vi "NML GPIB Data Log V1.00.vi"(0 "Point #":i32) -> (1 "GPIB Data":dbl[](array[numeric]) format="%.2e", 2 "Stop":bool)   [LabVIEW 2021]
doc: "VI which calls the appropriate GPIB routines for a variety of instruments.\nScott Hannahs, NHMFL-FSU, Nov. 1993"
uses:
  GPIB List.ctl
  Sub Controls/Instrument.ctl
  Sub Controls/NML GPIB List.ctl
panel:
  in  "Instrument":T1
  in  "Logcluster":T2 {"#1"."Parameters" format="%.3e"; "#5"."Parameters" format="%.3e"; "#3"."Parameters" format="%.3e"; "#2"."Parameters" format="%.3e"; "#4"."Parameters" format="%.3e"}
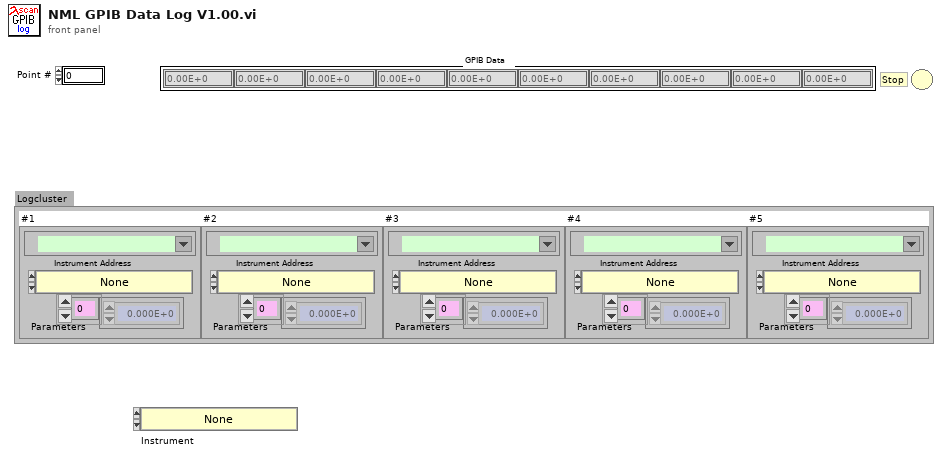
[diagram p1: front panel]
types:
  T1 = typedef "NML GPIB List.ctl" = enum16{"None", "Field", "Field - SCM1", "DMM", "DMM - HP 34401", "Keithley 2XXX", "Running DMM Ave", "Running HP34401", "Running K2XXX Ave", "SRS 830 - CH 1", "SRS 830 - CH1 & 2", "SRS PTC10", "Signal Rec 7265 - X", "Signal Rec 7265 - X&Y", "DRC 93C - Sample", "DRC 93C - Control", "DRC 93C - Sam&Con", "CryoCon Sensor A", "CryoCon Sensor B", "Cond 20C Sensor 1", "Cond 20C Sensor 2", "LS 336 Read", "LS 340 Read", "LS 370 Read", "LS 370 Select", "AVS 46 Bridge", "BLM Rotator Read Position", "Linear Research 700", "LR 700 Select", "Keithley 3330 - LCZ", "A-H Capacitance", "Digital Integrator", "SRS 400 Phot Ctr", "LakeShore VSM", "AMI He Level Meter", "Time Stamp", "Wait", "Invert Current", "K230 Linear V", "K230 VÅB^2", "Temp Ramp", "Power Ramp", "Freq Sweep", "LTC Stable T", "Scanner Step", "IMS Stepper Increment", "BLM Stepper Increment", "Omega CNi32"}
  T2 = typedef "GPIB List.ctl" = cluster{"#4":T3, "#2":T3, "#3":T3, "#5":T3, "#1":T3}
  T3 = typedef "Instrument.ctl" = cluster{"Instrument":T1, "Instrument Address":refnum<visa-resource-name>, "Parameters":dbl[]}
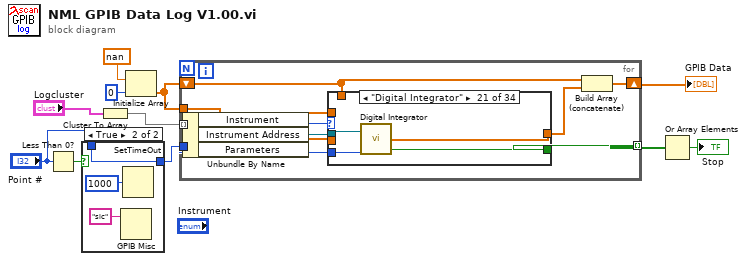
[diagram p0: block diagram]
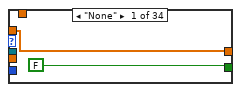
[diagram p3: hidden frame]
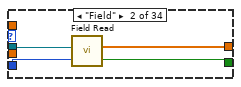
[diagram p4: hidden frame]
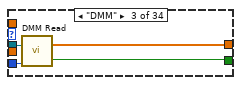
[diagram p5: hidden frame]
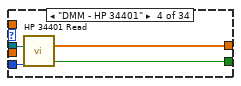
[diagram p6: hidden frame]
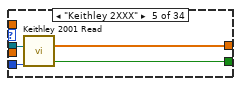
[diagram p7: hidden frame]
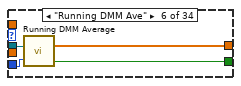
[diagram p8: hidden frame]
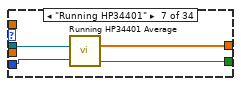
[diagram p9: hidden frame]
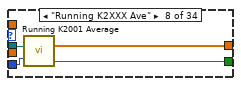
[diagram p10: hidden frame]
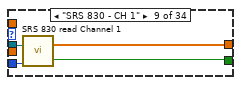
[diagram p11: hidden frame]
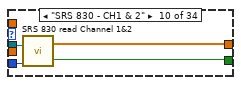
[diagram p12: hidden frame]
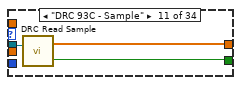
[diagram p13: hidden frame]
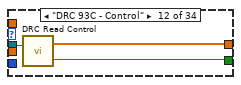
[diagram p14: hidden frame]
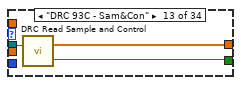
[diagram p15: hidden frame]
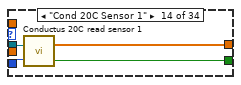
[diagram p16: hidden frame]
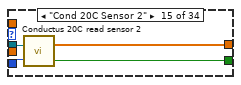
[diagram p17: hidden frame]
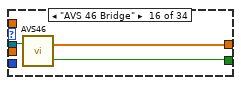
[diagram p18: hidden frame]
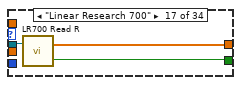
[diagram p19: hidden frame]
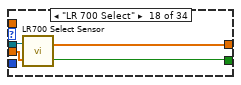
[diagram p20: hidden frame]
diagram:
  n1 = Less Than 0?(x="Point #") -> (x < 0?=w5:bool)
  n2 = case shown="True" w5 {
    tunnel: [w12 w14] -> w3
    tunnel: "Point #" -> [w12 w14]
    frame False {
    }
    frame True {
      n3 = GPIB Misc(0:"sic" ("command string")) -> ()  [unwired: 1 in, 3 out]
      n4 = SetTimeOut(1:1000 ("new timeout (10000)")) -> ()  [unwired: 1 out]
    }
  }
  n5 = Cluster To Array(cluster="Logcluster") -> (array=w1:T3[])
  n6 = Initialize Array(nan, 0) -> (w7:dbl[])
  n7 = for {
    shift-right: [w25] -> w11
    shift-left: w7 -> [w20]
    tunnel: w3 -> [w23]
    tunnel: [w22] -> w6 mode=indexing
    tunnel: w7 -> [w21]
    tunnel: w1 -> [w19] mode=indexing
    n8 = Unbundle By Name(w19) -> ("Instrument"=w16:T1, "Instrument Address"=w18:refnum<visa-resource-name>, "Parameters"=w17:dbl[])
    n9 = case shown="\"Digital Integrator\"" w16 {
      tunnel: [FALSE w30 w34 w38 w42 w46 w50 w54 w59 w63 w66 w69 w72 w75 w79 w82 w85 w89 w92 w96 w98 w104 w107 w109 w113 w118 w123 w128 w133 w138 w140 w146 w152 w154] -> w22
      tunnel: w23 -> [_ w28 w32 w36 w40 w44 w48 w52 w56 w60 _ _ _ w73 w77 _ _ _ _ w94 w101 _ _ w111 w115 w116 w120 w126 w131 w136 w142 w147 w151 w158]
      tunnel: [w26 w31 w35 w39 w43 w47 w51 w55 w58 w62 w65 w68 w71 w76 w80 w81 w84 w88 w91 w95 w99 w105 w108 w110 w114 w119 w124 w129 w134 w139 w141 w145 w153 w155] -> w24
      tunnel: w18 -> [_ w29 w33 w37 w41 w45 w49 w53 w57 w61 w64 w67 w70 w74 w78 w83 w86 w90 w93 w97 w100 w103 w106 _ _ w117 w122 w127 w132 w137 w143 w148 w150 w156]
      tunnel: w21 -> [w26 _ _ _ _ _ _ _ _ _ _ _ _ _ _ _ _ _ _ _ _ _ _ _ _ _ _ _ _ _ _ _ _ _]
      tunnel: w17 -> [_ _ _ _ _ _ _ _ _ _ _ _ _ _ _ _ _ w87 _ _ _ w102 _ _ w112 _ w121 _ w130 w135 _ w144 w149 w157]
      tunnel: w20 -> [_ _ _ _ _ _ _ _ _ _ _ _ _ _ _ _ _ _ _ _ _ _ _ _ _ _ _ w125 _ _ _ _ _ _]
      frame "None" {
      }
      frame "Field" {
        n10 = call "Field Read.vi"("Point #"=w28, "Instrument Address"=w29) -> ("Stop"=w30:bool, "Field"=w31:dbl[])
      }
      frame "DMM" {
        n11 = call "DMM Read.vi"("Point #"=w32, "Instrument Address"=w33) -> ("Stop"=w34:bool, "Measurement"=w35:dbl[])
      }
      frame "DMM - HP 34401" {
        n12 = call "HP 34401 Read.vi"("Point #"=w36, "Instrument Address"=w37) -> ("Stop"=w38:bool, "Measurement"=w39:dbl[])
      }
      frame "Keithley 2XXX" {
        n13 = call "Keithley 2001 Read.vi"("Point #"=w40, "Instrument Address"=w41) -> ("Stop"=w42:bool, "Measurement"=w43:dbl[])
      }
      frame "Running DMM Ave" {
        n14 = call "Running DMM Average.vi"("Point #"=w44, "Instrument Address"=w45) -> ("Stop"=w46:bool, 1:w47:dbl[])
      }
      frame "Running HP34401" {
        n15 = call "Running HP34401 Average.vi"("Point #"=w48, "Instrument Address"=w49) -> ("Stop"=w50:bool, 1:w51:dbl[])
      }
      frame "Running K2XXX Ave" {
        n16 = call "Running K2001 Average.vi"("Point #"=w52, "Instrument Address"=w53) -> ("Stop"=w54:bool, 1:w55:dbl[])
      }
      frame "SRS 830 - CH 1" {
        n17 = call "SRS 830 read Channel 1.vi"("Point #"=w56, "Instrument Address"=w57) -> ("Stop"=w59:bool, "SRS 830 Output"=w58:dbl[])
      }
      frame "SRS 830 - CH1 & 2" {
        n18 = call "SRS 830 read Channel 1&2.vi"("Point #"=w60, "Instrument Address"=w61) -> ("Stop"=w63:bool, "SRS 830 Output"=w62:dbl[])
      }
      frame "DRC 93C - Sample" {
        n19 = call "DRC Read Sample.vi"("Instrument Address"=w64) -> ("Stop"=w66:bool, "Output"=w65:dbl[])  [unwired: 1 in]
      }
      frame "DRC 93C - Control" {
        n20 = call "DRC Read Control.vi"("Instrument Address"=w67) -> ("Stop"=w69:bool, "Output"=w68:dbl[])  [unwired: 1 in]
      }
      frame "DRC 93C - Sam&Con" {
        n21 = call "DRC Read Sample and Control.vi"("Instrument Address"=w70) -> ("Stop"=w72:bool, "Output"=w71:dbl[])  [unwired: 1 in]
      }
      frame "Cond 20C Sensor 1" {
        n22 = call "Conductus 20C read sensor 1.vi"("Point #"=w73, "Instrument Address"=w74) -> ("Stop"=w75:bool, "Output"=w76:dbl[])
      }
      frame "Cond 20C Sensor 2" {
        n23 = call "Conductus 20C read sensor 2.vi"("Point #"=w77, "Instrument Address"=w78) -> ("Stop"=w79:bool, "Output"=w80:dbl[])
      }
      frame "AVS 46 Bridge" {
        n24 = call "AVS46.vi"("Instrument Address"=w83) -> ("Stop"=w82:bool, "Measurement"=w81:dbl[])  [unwired: 1 in]
      }
      frame "Linear Research 700" {
        n25 = call "LR700 Read R.vi"("Instrument Address"=w86) -> ("Stop"=w85:bool, "Measurement"=w84:dbl[])  [unwired: 1 in]
      }
      frame "LR 700 Select" {
        n26 = call "LR700 Select Sensor.vi"("Parameters"=w87, "Instrument Address"=w90) -> ("Stop"=w89:bool, "Array"=w88:dbl[])
      }
      frame "Keithley 3330 - LCZ" {
        n27 = call "Keithley 3330 Read.vi"("Instrument Address"=w93) -> ("Stop"=w92:bool, "Measurement"=w91:dbl[])  [unwired: 1 in]
      }
      frame "A-H Capacitance" {
        n28 = call "A-H Cap.vi"("Point #"=w94, "Instrument Address"=w97) -> ("Stop"=w96:bool, "Measurement"=w95:dbl[])
      }
      frame "Digital Integrator" {
        n29 = call "Digital Integrator.vi"("Instrument Address"=w100, "Index"=w101) -> (3:w99:dbl[], "Stop"=w98:bool)  [unwired: 1 out]
      }
      frame "SRS 400 Phot Ctr" {
        n30 = call "SRS 400 Read.vi"("Parameters"=w102, "Instrument Address"=w103) -> ("Stop"=w104:bool, "Data"=w105:dbl[])
      }
      frame "LakeShore VSM" {
        n31 = call "LakeShore VSM 7300 EMU read.vi"("Instrument Address"=w106) -> ("Stop"=w107:bool, "Output"=w108:dbl[])  [unwired: 1 in]
      }
      frame "Time Stamp" {
        n32 = call "Time Stamp-old.vi"("Point #"=w111) -> ("Stop"=w109:bool, "Time Stamp (Sec)"=w110:dbl[])  [unwired: 1 in]
      }
      frame "Wait" {
        n33 = call "Seconds Wait.vi"("Point #"=w115, "Parameters"=w112) -> ("Stop"=w113:bool, "Time Stamp (Sec)"=w114:dbl[])
      }
      frame "Invert Current" {
        n34 = call "Invert Current Keithley 220.vi"("Point #"=w116, "Instrument Address"=w117) -> ("Stop"=w118:bool, "Keithley 220 Current"=w119:dbl[])  [unwired: 2 in]
      }
      frame "K230 Linear V" {
        n35 = call "Keithley 230 Voltage Ramp.vi"("Point #"=w120, "Parameters"=w121, "Instrument Address"=w122) -> ("Stop"=w123:bool, "Keithley 230 Voltage"=w124:dbl[])  [unwired: 1 in]
      }
      frame "K230 VÅB^2" {
        n36 = call "Keithley 230 V prop B^2.vi"("Point #"=w126, "GPIB Data In"=w125, "Instrument Address"=w127) -> ("Stop"=w128:bool, "Keithley 230 Voltage"=w129:dbl[])  [unwired: 1 in]
      }
      frame "Temp Ramp" {
        n37 = call "Conductus Ramp Temperature.vi"("Point #"=w131, "Parameters"=w130, "Instrument Address"=w132) -> ("Stop"=w133:bool, "Data Out"=w134:dbl[])  [unwired: 1 in]
      }
      frame "Power Ramp" {
        n38 = call "Conductus Ramp Power.vi"("Point #"=w136, "Parameters"=w135, "Instrument Address"=w137) -> ("Stop"=w138:bool, "Data Out"=w139:dbl[])  [unwired: 1 in]
      }
      frame "LTC Stable T" {
        n39 = call "LTC change to stable temp.vi"("Point Number"=w142, "L:TC 21 Address"=w143) -> ("Stop"=w140:bool, "Stable temperature (K)"=w141:dbl[])
      }
      frame "Scanner Step" {
        n40 = call "Scanme.vi"("Index"=w147, "Parameters"=w144, "Instrument Address"=w148) -> ("Stop"=w146:bool, "Array"=w145:dbl[])  [unwired: 1 in]
      }
      frame "IMS Stepper Increment" {
        n41 = call "Parker Stepper Control.vi"("Point #"=w151, "Parameters"=w149, "Instrument Address"=w150) -> ("Stop"=w152:bool, "Data Out"=w153:dbl[])  [unwired: 1 in]
      }
      frame "BLM Stepper Increment", Default {
        n42 = call "Parker Stepper Client.vi"("Point #"=w158, "Parameters"=w157, "Port"=w156) -> ("Stop"=w154:bool, "Data Out"=w155:dbl[])  [unwired: 1 in]
      }
    }
    n43 = Build Array (concatenate)(w20, w24) -> (w25:dbl[])
  }
  "GPIB Data" <- w11
  n44 = Or Array Elements(Boolean array=w6) -> (logical OR=→"Stop":bool)
